vi "HXG2enableFGV.vi"(6 "LIQ EN":refnum<vi>, 7 "ENABLE Ctrl":T1=enum."Write", 8 "error in (no error)":errorcluster, 9 "Air EN":refnum<vi>, 10 "LIQ EN":bool, 11 "Air EN":bool) -> (0 "error out":errorcluster, 2 "Air-Liq Refs":refnum<vi>[](array[refnum]), 3 "Air-Liq Out":bool[](array[boolean]))   [LabVIEW 2012]
doc: "Gets, Sets and Resets the state of the AIR ENABLE BUTTON"
uses:
  HXG2enable.ctl
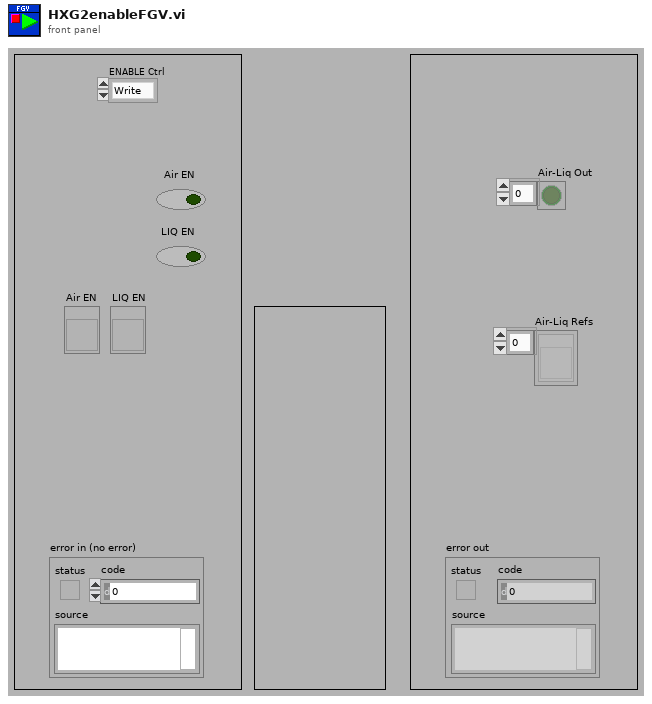
[diagram p1: front panel]
types:
  T1 = typedef "HXG2enable.ctl" = enum16{"Write Refs", "Write", "Pass"}
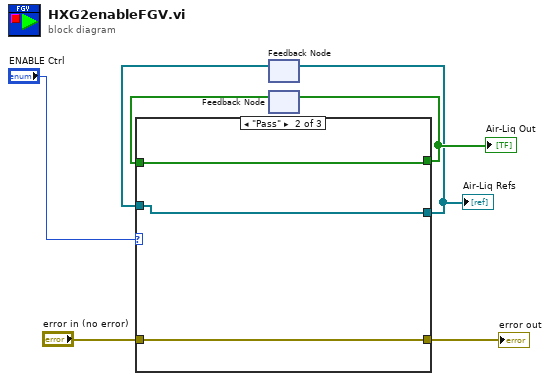
[diagram p0: block diagram]
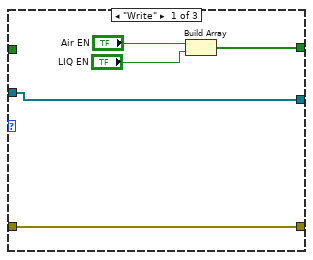
[diagram p2: hidden frame]
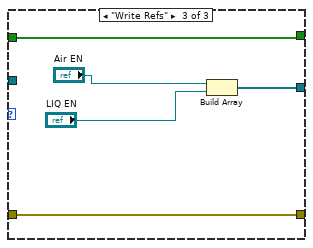
[diagram p3: hidden frame]
diagram:
  n1 = feedback #1() -> (w1:refnum<vi>[])  [unwired: 1 in]
  n2 = feedback #2() -> (w7:bool[])  [unwired: 1 in]
  n3 = case shown="\"Pass\"" "ENABLE Ctrl" {
    tunnel: [w11 w14 w18] -> w4
    tunnel: w7 -> [_ w14 w18]
    tunnel: "error in (no error)" -> [w12 w15 w20]
    tunnel: [w12 w15 w20] -> w5
    tunnel: [w8 w13 w19] -> w2
    tunnel: w1 -> [w8 w13 _]
    frame "Write" {
      n4 = Build Array("Air EN", "LIQ EN") -> (w11:bool[])
    }
    frame "Pass" {
    }
    frame "Write Refs" {
      n5 = Build Array("Air EN", "LIQ EN") -> (w19:refnum<vi>[])
    }
  }
  "error out" <- w5
  "Air-Liq Refs" <- w2
  "Air-Liq Out" <- w4
  n6 = feedback-in #1(w2) -> ()
  n7 = feedback-in #2(w4) -> ()
